vi "database_connection_write_DMMS.vi"(5 "ODBC data source name":string="amrc_monitoring", 6 "error in (no error)":errorcluster, 7 "G1?":u32, 8 "current time":timestamp, 9 "data 2":dbl[](array[numeric]), 10 "Machine Data":T1={"Zload"="", "Yload"="", "Xload"="", "path_position"="", "Fovr"="", "SspeedOvr"="", "Program Name"="", "Program status"="", "Block of code being executed"="", "Line of code"="", "Machine availability"="", "Emergency status"="", "Controller mode"="", "Tool_id"="UNAVAILABLE"}, 11 "Machine type":string) -> (3 "error out":errorcluster)   [LabVIEW 2017]
uses:
  <vilib>/addons/database/Connection.llb/DB Tools Open Connec (String).vi
  <vilib>/addons/database/Connection.llb/Conn Execute.vi
  <vilib>/addons/database/Recordset.llb/Rec Destroy - Connection.vi
  <vilib>/addons/database/Connection.llb/DB Tools Open Connec (Path).vi
  <vilib>/addons/database/NI_Database_API.lvlib
panel:
  out "error out 2":errorcluster
  out "Tool_id":string
  out "resulting string":string
  out "size(s)":i32
  out "concatenated string 5":string
  out "concatenated string 4":string
  out "concatenated string 3":string
  out "concatenated string 2":string
  out "concatenated string":string
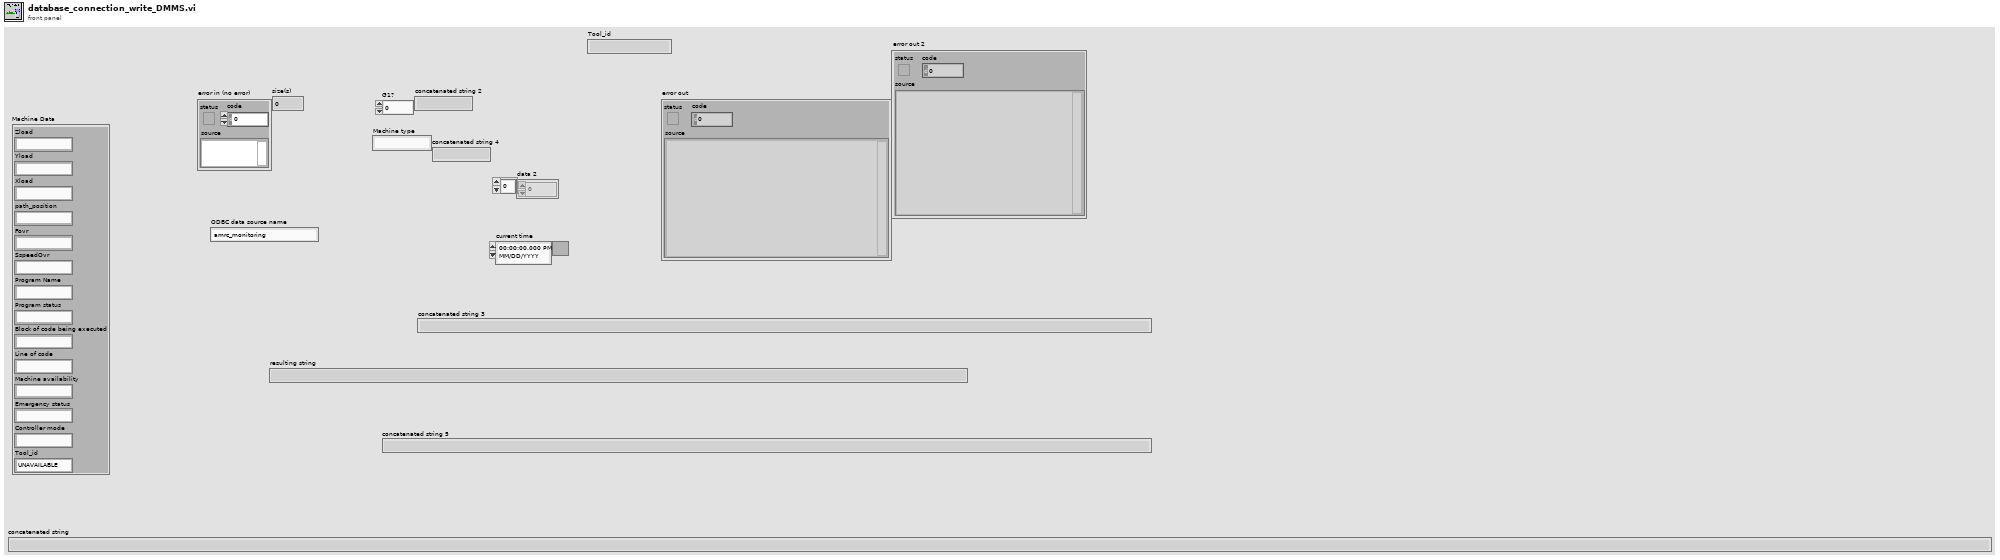
[diagram p1: front panel]
types:
  T1 = cluster{"Zload":string, "Yload":string, "Xload":string, "path_position":string, "Fovr":string, "SspeedOvr":string, "Program Name":string, "Program status":string, "Block of code being executed":string, "Line of code":string, "Machine availability":string, "Emergency status":string, "Controller mode":string, "Tool_id":string}
  T2 = typedef "NI_Database_API.lvlib/Conn ObjectReference.ctl" = refnum<k1>
  T3 = typedef "NI_Database_API.lvlib/Rec ObjectReference.ctl" = refnum<k1>
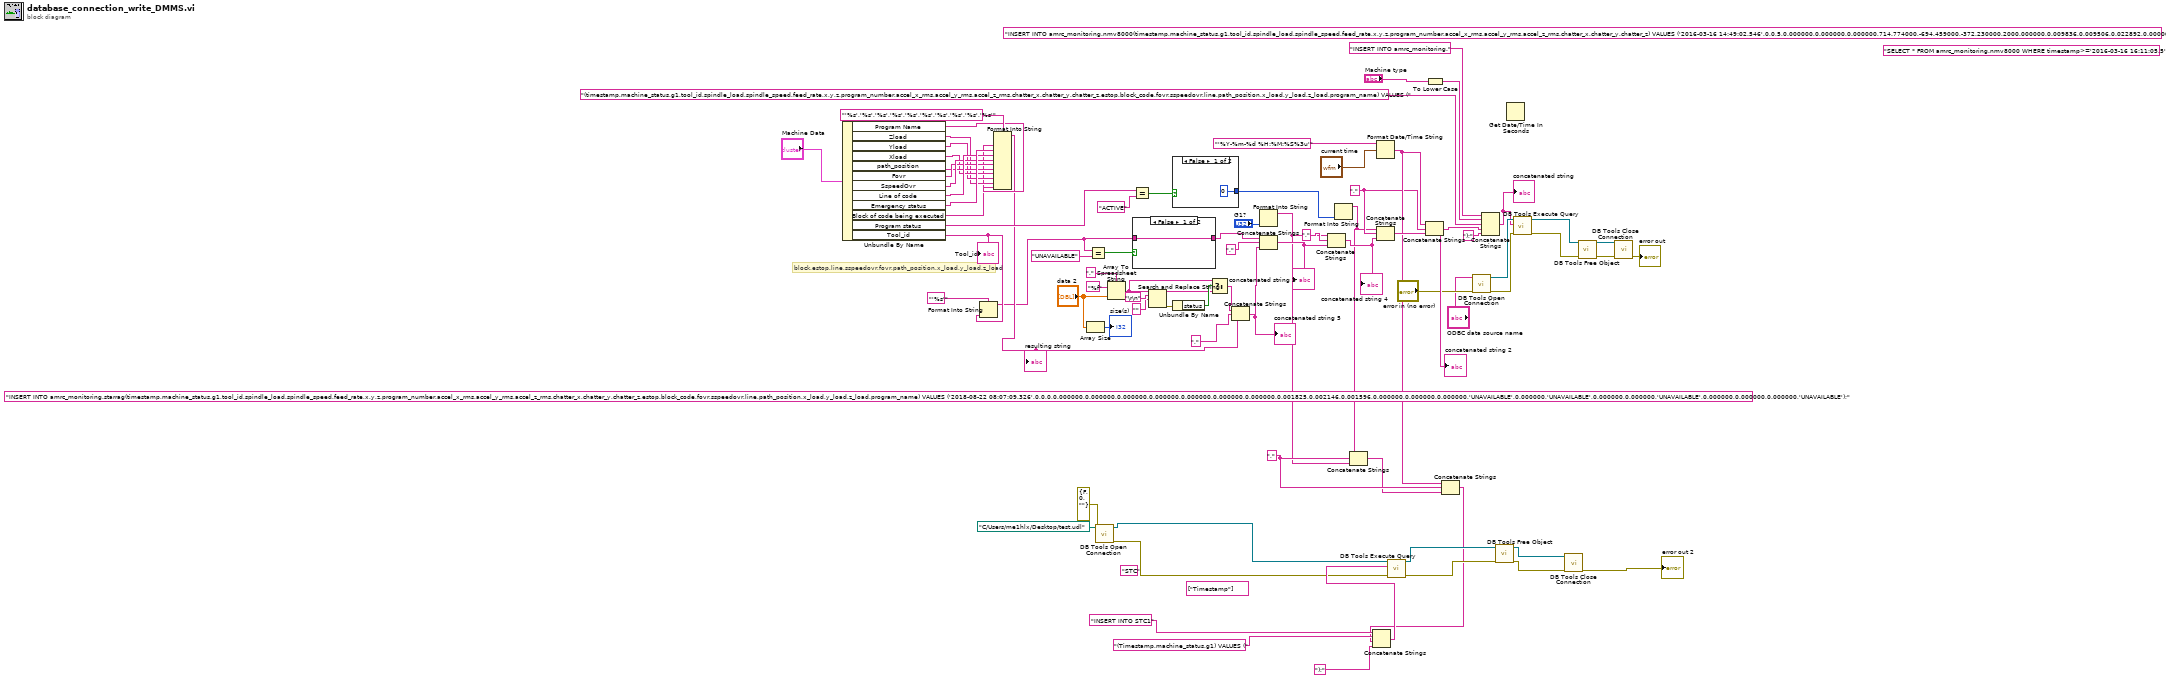
[diagram p0: block diagram]
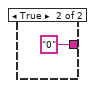
[diagram p2: hidden frame]
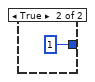
[diagram p3: hidden frame]
diagram:
  w16 = "," ("string")
  (unwired) string[] ["Timestamp"]
  (unwired) "STC"
  (unwired) "INSERT INTO amrc_monitoring.starrag(timestamp,machine_status,g1,tool_id,spindle_load,spindle_speed,feed_rate,x,y,z,program_number,accel_x_rms,accel_y_rms,accel_z_rms,chatter_x,chatter_y,chatter_z,estop,block_code,fovr,sspeedovr,line,path_position,x_load,y_load,z_load,program_name) VALUES ('2018-08-22 08:07:09.326',0,0,0,0.000000,0.000000,0.000000,0.000000,0.000000,0.000000,0.000000,0.001825,0.002146,0.001596,0.000000,0.000000,0.000000,'UNAVAILABLE',0.000000,'UNAVAILABLE',0.000000,0.000000,'UNAVAILABLE',0.000000,0.000000,0.000000,'UNAVAILABLE');" ("string")
  w18 = "," ("string")
  (unwired) "SELECT * FROM amrc_monitoring.nmv8000 WHERE timestamp>='2016-03-16 16:11:05.5' " ("SQL query")
  (unwired) "INSERT INTO amrc_monitoring.nmv8000(timestamp,machine_status,g1,tool_id,spindle_load,spindle_speed,feed_rate,x,y,z,program_number,accel_x_rms,accel_y_rms,accel_z_rms,chatter_x,chatter_y,chatter_z) VALUES ('2016-03-16 14:49:02.546',0,0,5,0.000000,0.000000,0.000000,714.774000,-694.459000,-372.230000,2000.000000,0.009836,0.009506,0.022892,0.000000,1.000000,0.000000);" ("SQL query")
  # "block,estop,line,sspeedovr,fovr,path_position,x_load,y_load,z_load"
  n1 = Unbundle By Name("Machine Data") -> ("Program Name"=w36:string, "Zload"=w41:string, "Yload"=w42:string, "Xload"=w43:string, "path_position"=w44:string, "Fovr"=w45:string, "SspeedOvr"=w46:string, "Line of code"=w47:string, "Emergency status"=w48:string, "Block of code being executed"=w33:string, "Program status"=w73:string, "Tool_id"=w23:string)
  "Tool_id" <- w23
  n2 = Format Into String(format string="'%s'", w23) -> (resulting string=w22:string)  [unwired: 2 in, 1 out]
  n3 = Format Into String(format string="'%s','%s','%s','%s','%s','%s','%s','%s','%s','%s'", w33, w48, w47, w46, w45, w44, w43, w42, w41, w36) -> (resulting string=w27:string)  [unwired: 2 in, 1 out]
  "resulting string" <- w27
  n4 = Array Size(array="data 2") -> (size(s)=→"size(s)":i32)
  n5 = Equal?(x=w22, y="UNAVAILABLE") -> (x = y?=w69:bool)
  n6 = call-poly <vilib>:"DB Tools Open Connection.vi"("error in (no error)"=errorcluster {"status"=FALSE, "code"=0, "source"=""}, "connection information"=path "C:/Users/me1hlx/Desktop/test.udl") -> ("error out"=w10:errorcluster, "connection reference"=w1:T2)  [unwired: 6 in]
  n7 = Array To Spreadsheet String(delimiter (Tab)=",", array="data 2", 3:"%f" ("format string")) -> (spreadsheet string=w58:string)
  n8 = case shown="False" w69 {
    tunnel: w22 -> [w81 _]
    tunnel: [w81 "0"] -> w25
    frame False {
    }
    frame True {
    }
  }
  n9 = Equal?(x=w73, y="ACTIVE") -> (x = y?=w71:bool)
  n10 = Search and Replace String(input string=w58, search string="\r\n", replace string="" ("replace string (\"\")")) -> (result string=w59:string, error out=w61:errorcluster)  [unwired: 5 in, 2 out]
  n11 = case shown="False" w71 {
    tunnel: [0 1] -> w70
    frame False {
    }
    frame True {
    }
  }
  n12 = Unbundle By Name(w61) -> ("status"=w60:bool)
  n13 = Select(t=w58, s=w60, f=w59) -> (s? t:f=w38:string)
  n14 = Concatenate Strings(w38, "," ("string"), w27) -> (w37:string)
  "concatenated string 5" <- w37
  n15 = Format Into String("G1?") -> (resulting string=w13:string)  [unwired: 3 in, 1 out]
  n16 = Concatenate Strings(w25, "," ("string"), w37) -> (w31:string)
  "concatenated string 3" <- w31
  n17 = Concatenate Strings(w13, "," ("string"), w31) -> (w17:string)
  "concatenated string 4" <- w17
  n18 = Format Into String(w70) -> (resulting string=w15:string)  [unwired: 3 in, 1 out]
  n19 = Concatenate Strings(w15, w16, w13) -> (w14:string)
  n20 = Concatenate Strings(w15, w18, w17) -> (w65:string)
  n21 = Format Date/Time String(time format string (%c)="'%Y-%m-%d %H:%M:%S%3u'", seconds (now)="current time") -> (date/time string=w19:string)  [unwired: 1 in]
  n22 = Concatenate Strings(w19, w18, w65) -> (w64:string)
  "concatenated string 2" <- w64
  n23 = To Lower Case(string="Machine type") -> (all lower case string=w55:string)
  n24 = Concatenate Strings(w19, w16, w14) -> (w2:string)
  n25 = Concatenate Strings("INSERT INTO STC1" ("string"), "(Timestamp,machine_status,g1) VALUES (" ("string"), w2, ");" ("string")) -> (w11:string)
  n26 = call-poly <vilib>:"DB Tools Execute Query.vi"("error in (no error)"=w10, "SQL query"=w11, "connection reference"=w1) -> ("error out"=w7:errorcluster, "recordset reference"=w8:T3)  [unwired: 5 in]
  n27 = call-poly <vilib>:"DB Tools Open Connection.vi"("error in (no error)"="error in (no error)", "connection information"="ODBC data source name") -> ("error out"=w79:errorcluster, "connection reference"=w80:T2)  [unwired: 6 in]
  n28 = Concatenate Strings("INSERT INTO amrc_monitoring." ("string"), w55, "(timestamp,machine_status,g1,tool_id,spindle_load,spindle_speed,feed_rate,x,y,z,program_number,accel_x_rms,accel_y_rms,accel_z_rms,chatter_x,chatter_y,chatter_z,estop,block_code,fovr,sspeedovr,line,path_position,x_load,y_load,z_load,program_name) VALUES (" ("string"), w64, ");" ("string")) -> (w28:string)
  "concatenated string" <- w28
  n29 = call-poly <vilib>:"DB Tools Free Object.vi"("error in (no error)"=w7, "recordset reference"=w8) -> ("error out"=w5:errorcluster, "connection reference"=w6:T2)  [unwired: 8 in]
  n30 = Get Date/Time In Seconds() -> ()  [unwired: 1 out]
  n31 = call-poly <vilib>:"DB Tools Execute Query.vi"("error in (no error)"=w79, "SQL query"=w28, "connection reference"=w80) -> ("error out"=w51:errorcluster, "recordset reference"=w50:T3)  [unwired: 5 in]
  n32 = call <vilib>:"DB Tools Close Connection.vi"("error in (no error)"=w5, "connection reference"=w6) -> ("error out"=→"error out 2":errorcluster)  [unwired: 5 in]
  n33 = call-poly <vilib>:"DB Tools Free Object.vi"("error in (no error)"=w51, "recordset reference"=w50) -> ("error out"=w78:errorcluster, "connection reference"=w77:T2)  [unwired: 8 in]
  n34 = call <vilib>:"DB Tools Close Connection.vi"("error in (no error)"=w78, "connection reference"=w77) -> ("error out"=→"error out":errorcluster)  [unwired: 5 in]
